vi "RingToEnum.vi"(10 "Numeric":u16, 11 "Enum":variant) -> (2 "Value":i32)   [LabVIEW 2011]
uses:
  LVStringsAndValuesArrayTypeDef.ctl
panel:
  out "Enum Name":string
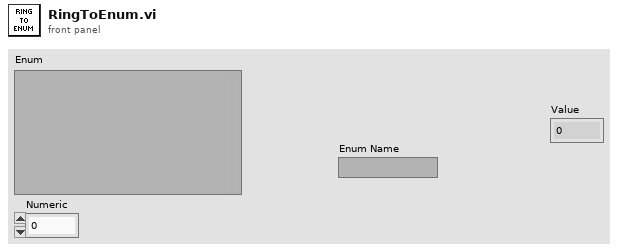
[diagram p1: front panel]
types:
  T1 = typedef "LVStringsAndValuesArrayTypeDef.ctl" = cluster{"String":string, "Value":ext}[]
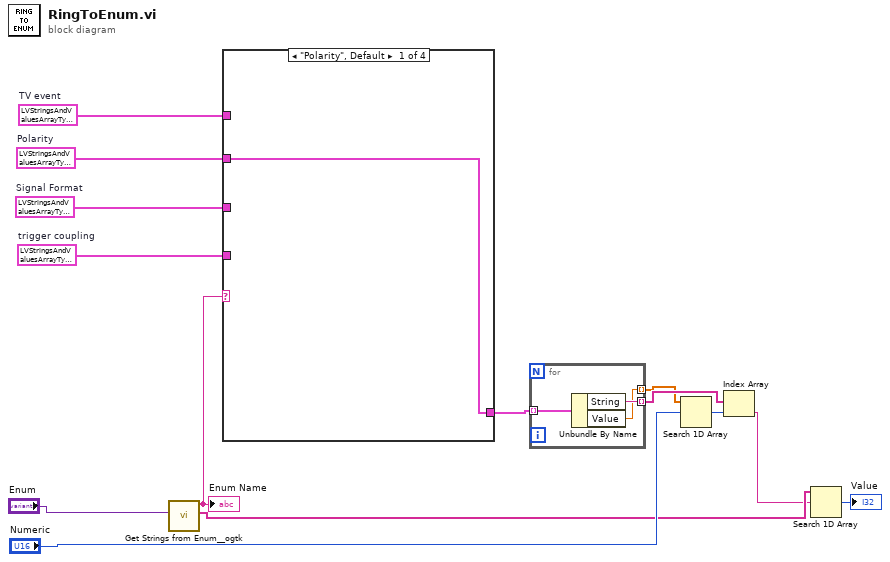
[diagram p0: block diagram]
diagram:
  w12 = T1 [{"String"="M-NTSC", "Value"=1.0}, {"String"="B/G-PAL", "Value"=2.0}, {"String"="SECAM", "Value"=3.0}, {"String"="M-PAL", "Value"=1001.0}, {"String"="480i/59.94 fps", "Value"=1010.0}, {"String"="480i/60 fps", "Value"=1011.0}, {"String"="480p/59.94 Fps", "Value"=1015.0}, {"String"="480p/60 Fps", "Value"=1016.0}, {"String"="576i/50 fps", "Value"=1020.0}, {"String"="576p/50 Fps", "Value"=1025.0}, {"String"="720p/50 Fps", "Value"=1031.0}, {"String"="720p/59.94 Fps", "Value"=1032.0}, {"String"="720p/60 Fps", "Value"=1033.0}, {"String"="1080i/50 fps", "Value"=1040.0}, {"String"="1080i/59.94 fps", "Value"=1041.0}, {"String"="1080i/60 fps", "Value"=1042.0}, {"String"="1080p/24 Fps", "Value"=1045.0}]  # Signal Format
  w9 = T1 [{"String"="Field 1", "Value"=1.0}, {"String"="Field 2", "Value"=2.0}, {"String"="Any Field", "Value"=3.0}, {"String"="Any Line", "Value"=4.0}, {"String"="Line Number", "Value"=5.0}]  # TV event
  w10 = T1 [{"String"="Positive", "Value"=1.0}, {"String"="Negative", "Value"=2.0}]  # Polarity
  w8 = T1 [{"String"="AC", "Value"=0.0}, {"String"="DC", "Value"=1.0}, {"String"="HF Reject", "Value"=3.0}, {"String"="LF Reject", "Value"=4.0}, {"String"="AC Plus HF Reject", "Value"=1001.0}]  # trigger coupling
  n1 = call "Get Strings from Enum__ogtk.vi"("Enum"="Enum") -> ("Enum Strings"=w3:string[], "Enum Name"=w13:string)  [unwired: 7 in, 2 out]
  "Enum Name" <- w13
  n2 = case shown="\"Polarity\", Default" w13 {
    tunnel: w12 -> [_ _ _ w18]
    tunnel: [w15 w16 w17 w18] -> w11
    tunnel: w10 -> [w15 _ _ _]
    tunnel: w9 -> [_ w16 _ _]
    tunnel: w8 -> [_ _ w17 _]
    frame "Polarity", Default {
    }
    frame "TV Event" {
    }
    frame "Coupling" {
    }
    frame "Signal Format" {
    }
  }
  n3 = for {
    tunnel: w11 -> [w21] mode=indexing
    tunnel: [w20] -> w6 mode=indexing
    tunnel: [w19] -> w5 mode=indexing
    n4 = Unbundle By Name(w21) -> ("String"=w20:string, "Value"=w19:ext)
  }
  n5 = Search 1D Array(1D array=w5, element="Numeric") -> (index of element=w14:i32)  [unwired: 1 in]
  n6 = Index Array(array=w6, index=w14) -> (element=w2:string)
  n7 = Search 1D Array(1D array=w3, element=w2) -> (index of element=→"Value":i32)  [unwired: 1 in]
